vi "Gpio.vi"() -> ()   [LabVIEW 2023, in "Numato.lvlib"]
uses:
  Numato.lvlib
  d040eff6-5516-4aa1-b987-fa9779415414.vi
panel:
  out "data out":string
  out "error out":errorcluster
  in  "error in (no error)":errorcluster
  in  "remote port or service name":u16=23
  in  "address":string
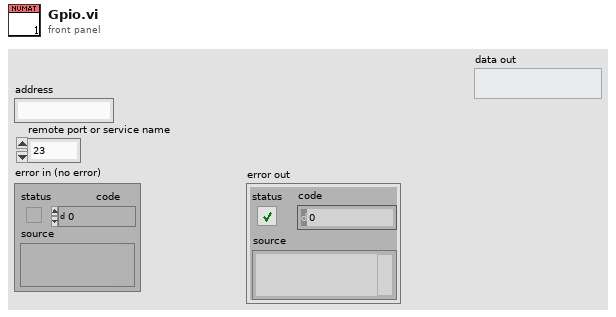
[diagram p1: front panel]
types:
  T1 = enum16{"Standard", "Buffered", "CRLF", "Immediate"}
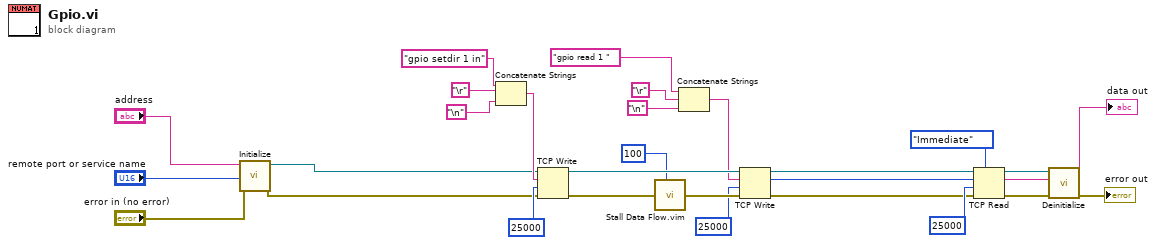
[diagram p0: block diagram]
diagram:
  n1 = call "Initialize.vi"("error in (no error)"="error in (no error)", "remote port or service name"="remote port or service name", "address"="address") -> ("error out"=w1:errorcluster, "connection ID out"=w2:refnum<k5>)  [unwired: 6 in]
  n2 = Concatenate Strings("gpio setdir 1 in" ("data in"), "\r", "\n") -> (w14:string)
  n3 = TCP Write(connection ID=w2, data in=w14, error in (no error)=w1, 9:25000 ("timeout ms (25000)")) -> (connection ID out=w19:refnum<k5>, error out=w17:errorcluster)  [unwired: 1 out]
  n4 = call "Stall Data Flow.vim"("value in"=w17, "milliseconds to wait"=u32 100) -> ("value out"=w18:errorcluster)  [unwired: 1 out]
  n5 = Concatenate Strings("gpio read 1 " ("data in"), "\r", "\n") -> (w10:string)
  n6 = TCP Write(connection ID=w19, data in=w10, error in (no error)=w18, 9:25000 ("timeout ms (25000)")) -> (connection ID out=w5:refnum<k5>, bytes written=w3:i32, error out=w4:errorcluster)
  n7 = TCP Read(connection ID=w5, bytes to read=w3, error in (no error)=w4, 7:T1."Immediate" ("mode (standard)"), 9:25000 ("timeout ms (25000)")) -> (connection ID out=w24:refnum<k5>, data out=→"data out":string, error out=w23:errorcluster)
  n8 = call "Deinitialize.vi"("error in (no error)"=w23, "connection ID"=w24) -> ("error out"=→"error out":errorcluster)  [unwired: 9 in]
